vi "Load.vi"(8 "error in (no error)":errorcluster) -> (0 "error out":errorcluster, 3 "App Config Data Out":T1)   [LabVIEW 2015, in "App Config.lvlib"]
uses:
  App Config.lvlib
  App Config Data.ctl
  <vilib>/Utility/xml.llb/Read From XML File(string).vi
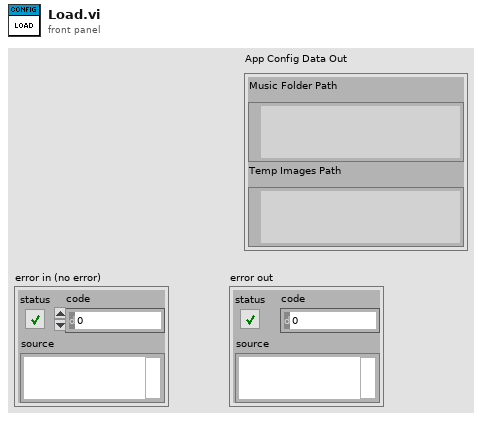
[diagram p1: front panel]
types:
  T1 = typedef "App Config.lvlib/App Config Data.ctl" = cluster{"Music Folder Path":path, "Temp Images Path":path}
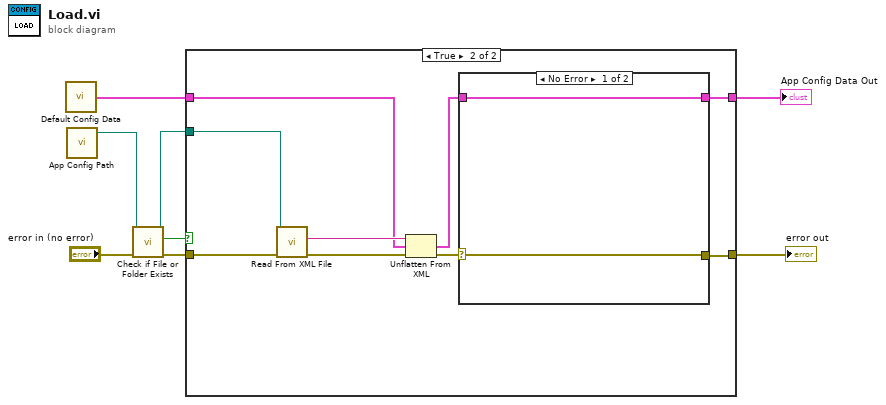
[diagram p0: block diagram]
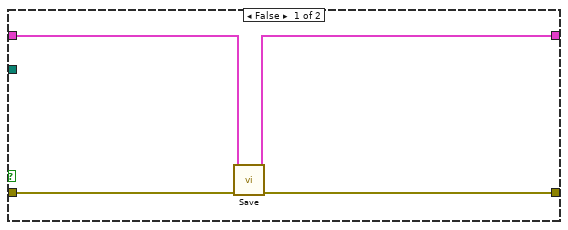
[diagram p2: hidden frame]
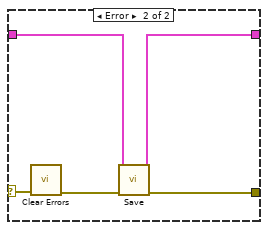
[diagram p3: hidden frame]
diagram:
  n1 = call "Default Config Data.vi"() -> ("Default Data"=w1:T1)  [unwired: 5 in]
  n2 = call "App Config Path.vi"() -> ("App Config Path"=w7:path)  [unwired: 5 in]
  n3 = call <vilib>:"Check if File or Folder Exists.vi"("error in (no error)"="error in (no error)", "path"=w7) -> ("error out"=w6:errorcluster, "file or folder exists?"=w5:bool, "dup path"=w4:path)  [unwired: 7 in]
  n4 = case shown="True" w5 {
    tunnel: w6 -> [w12 w21]
    tunnel: w4 -> [_ w20]
    tunnel: w1 -> [w10 w17]
    tunnel: [w11 w13] -> w3
    tunnel: [w9 w15] -> w2
    frame False {
      n5 = call "Save.vi"("error in (no error)"=w12, "App Config Data In"=w10) -> ("error out"=w11:errorcluster, "App Config Data Out"=w9:T1)  [unwired: 8 in]
    }
    frame True {
      n6 = call-poly <vilib>:"Read From XML File.vi"("error in (no error)"=w21, "XML File Path"=w20) -> ("error out"=w19:errorcluster, "XML Elements"=w18:string)  [unwired: 7 in, 1 out]
      n7 = Unflatten From XML(xml string=w18, type=w17, error in (no error)=w19) -> (value=w14:T1, error out=w16:errorcluster)
      n8 = case shown="No Error" w16 {
        selector: w16 -> [w22 w28]
        tunnel: [w23 w25] -> w15
        tunnel: w14 -> [w23 w26]
        tunnel: [w22 w24] -> w13
        frame No Error {
        }
        frame Error {
          n9 = call <vilib>:"Clear Errors.vi"("error in (no error)"=w28) -> ("error out"=w27:errorcluster)  [unwired: 5 in, 1 out]
          n10 = call "Save.vi"("error in (no error)"=w27, "App Config Data In"=w26) -> ("error out"=w24:errorcluster, "App Config Data Out"=w25:T1)  [unwired: 8 in]
        }
      }
    }
  }
  "error out" <- w3
  "App Config Data Out" <- w2
